vi "Measure Waveform.vi"(6 "Target Data":T1, 8 "error in (no error)":errorcluster, 9 "Measurement":T3, 10 "Channel":T2, 11 "MSOX6004 in":refnum<class "MSOX6004.lvclass">) -> (0 "error out":errorcluster, 2 "Measurement":dbl, 3 "MSOX6004 out":refnum<class "MSOX6004.lvclass">)   [LabVIEW 2018, in "MSOX6004.lvlib" / "MSOX6004.lvclass"]
uses:
  MSOX6004.lvclass
  PPLs/Oscilloscope/Parent/Oscilloscope.lvlibp/Custom Controls/Measurement.ctl
  PPLs/Oscilloscope/Parent/Oscilloscope.lvlibp/Custom Controls/Analog Channels.ctl
  PPLs/Oscilloscope/Parent/Oscilloscope.lvlibp/Custom Controls/Target Data.ctl
  MSOX6004.lvclass/MSOX6004.ctl
  <instrlib>/Keysight InfiniiVision/Keysight InfiniiVision.lvlib
  PPLs/Oscilloscope/Parent/Oscilloscope.lvlibp
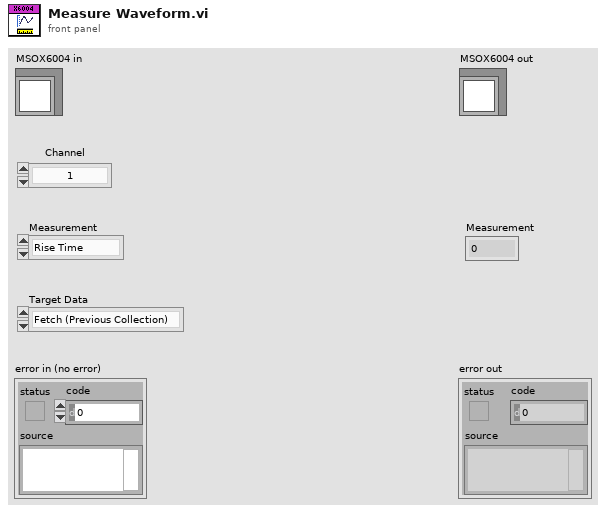
[diagram p1: front panel]
types:
  T1 = typedef "Oscilloscope.lvlibp/Target Data.ctl" = enum16{"Fetch (Previous Collection)", "Measure (New Collection)"}
  T2 = typedef "Oscilloscope.lvlibp/Analog Channels.ctl" = enum16{"1", "2", "3", "4", "5", "6", "7", "8", "9", "10", "11", "12", "13", "14", "15", "16"}
  T3 = typedef "Oscilloscope.lvlibp/Measurement.ctl" = enum16{"Rise Time", "Fall Time", "Frequency", "Period", "RMS (V)", "Peak-Peak (V)", "Max (V)", "Min (V)", "High State (V)", "Low State (V)", "Average (V)", "Width (Negative)", "Width (Positive)", "Duty Cycle (Negative)", "Duty Cycle (Positive)", "Amplitude", "Cycle RMS (V)", "Cycle Avg (V)", "Overshoot", "Preshoot", "Time at Max", "Frequency Counter", "Time at Min", "Delay", "Value at Time", "Phase", "Time at Value", "Time of Edge", "Area", "Burst Width", "Falling Edge Count", "Rising Edge Count", "Falling Pulse Count", "Rising Pulse Count", "Std Dev", "Pulse Width"}
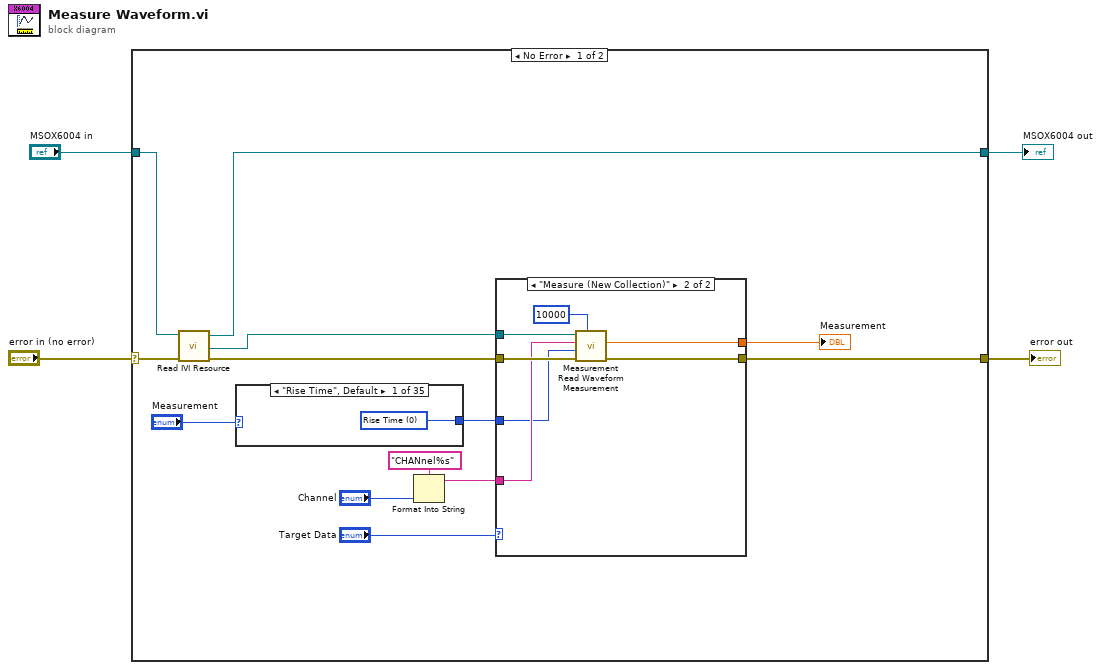
[diagram p0: block diagram]
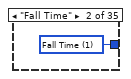
[diagram p2: hidden frame]
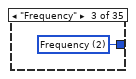
[diagram p3: hidden frame]
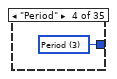
[diagram p4: hidden frame]
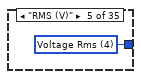
[diagram p5: hidden frame]
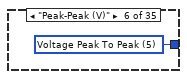
[diagram p6: hidden frame]
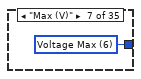
[diagram p7: hidden frame]
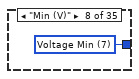
[diagram p8: hidden frame]
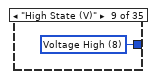
[diagram p9: hidden frame]
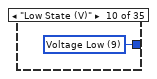
[diagram p10: hidden frame]
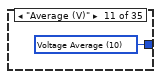
[diagram p11: hidden frame]
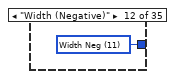
[diagram p12: hidden frame]
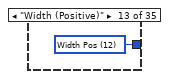
[diagram p13: hidden frame]
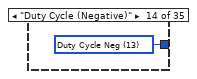
[diagram p14: hidden frame]
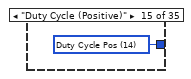
[diagram p15: hidden frame]
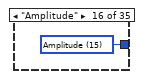
[diagram p16: hidden frame]
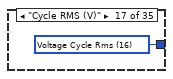
[diagram p17: hidden frame]
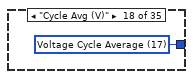
[diagram p18: hidden frame]
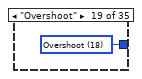
[diagram p19: hidden frame]
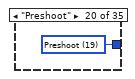
[diagram p20: hidden frame]
diagram:
  n1 = case shown="No Error" "error in (no error)" {
    selector: "error in (no error)" -> [w17 w67]
    tunnel: [w12 w67] -> w3
    tunnel: [w15 w66] -> w2
    tunnel: "MSOX6004 in" -> [w16 w66]
    frame No Error {
      n2 = call "Read IVI Resource.vi"("error in (no error)"=w17, "MSOX6004 in"=w16) -> ("error out"=w13:errorcluster, "IVI Resource"=w10:refnum<k15>, "MSOX6004 out"=w15:refnum<class "MSOX6004.lvclass">)  [unwired: 7 in]
      n3 = case shown="\"Rise Time\", Default" "Measurement" {
        tunnel: [w18 w19 w20 w21 w22 w23 w24 w25 w26 w27 w28 w29 w30 w31 w32 w33 w34 w35 w36 w37 w38 w39 w40 w41 w42 w43 w44 w45 w46 w47 w48 w49 w50 w51 w52] -> w5
        frame "Rise Time", Default {
          w18 = 0 items=["Rise Time"=0, "Fall Time"=1, "Frequency"=2, "Period"=3, "Voltage Rms"=4, "Voltage Peak To Peak"=5, "Voltage Max"=6, "Voltage Min"=7, "Voltage High"=8, "Voltage Low"=9, "Voltage Average"=10, "Width Neg"=11, "Width Pos"=12, "Duty Cycle Neg"=13, "Duty Cycle Pos"=14, "Amplitude"=15, "Voltage Cycle Rms"=16, "Voltage Cycle Average"=17, "Overshoot"=18, "Preshoot"=19, "Measurement Time At Max"=21, "Measurement Frequency Counter"=20, "Measurement Time At Min"=22, "Measurement Delay"=23, "Measurement Value At Time"=25, "Measurement Phase"=24, "Measurement Time At Value"=26, "Measurement Time Of Edge"=27, "Measurement Area"=28, "Measurement Burst Width"=29, "Measurement Falling Edge Count"=30, "Measurement Rising Edge Count"=32, "Measurement Falling Pulse Count"=31, "Measurement Rising Pulse Count"=33, "Measurement Standard Deviation"=34] ("MeasFunction (Rise Time)")
        }
        frame "Fall Time" {
          w19 = 1 items=["Rise Time"=0, "Fall Time"=1, "Frequency"=2, "Period"=3, "Voltage Rms"=4, "Voltage Peak To Peak"=5, "Voltage Max"=6, "Voltage Min"=7, "Voltage High"=8, "Voltage Low"=9, "Voltage Average"=10, "Width Neg"=11, "Width Pos"=12, "Duty Cycle Neg"=13, "Duty Cycle Pos"=14, "Amplitude"=15, "Voltage Cycle Rms"=16, "Voltage Cycle Average"=17, "Overshoot"=18, "Preshoot"=19, "Measurement Time At Max"=21, "Measurement Frequency Counter"=20, "Measurement Time At Min"=22, "Measurement Delay"=23, "Measurement Value At Time"=25, "Measurement Phase"=24, "Measurement Time At Value"=26, "Measurement Time Of Edge"=27, "Measurement Area"=28, "Measurement Burst Width"=29, "Measurement Falling Edge Count"=30, "Measurement Rising Edge Count"=32, "Measurement Falling Pulse Count"=31, "Measurement Rising Pulse Count"=33, "Measurement Standard Deviation"=34] ("MeasFunction (Rise Time)")
        }
        frame "Frequency" {
          w20 = 2 items=["Rise Time"=0, "Fall Time"=1, "Frequency"=2, "Period"=3, "Voltage Rms"=4, "Voltage Peak To Peak"=5, "Voltage Max"=6, "Voltage Min"=7, "Voltage High"=8, "Voltage Low"=9, "Voltage Average"=10, "Width Neg"=11, "Width Pos"=12, "Duty Cycle Neg"=13, "Duty Cycle Pos"=14, "Amplitude"=15, "Voltage Cycle Rms"=16, "Voltage Cycle Average"=17, "Overshoot"=18, "Preshoot"=19, "Measurement Time At Max"=21, "Measurement Frequency Counter"=20, "Measurement Time At Min"=22, "Measurement Delay"=23, "Measurement Value At Time"=25, "Measurement Phase"=24, "Measurement Time At Value"=26, "Measurement Time Of Edge"=27, "Measurement Area"=28, "Measurement Burst Width"=29, "Measurement Falling Edge Count"=30, "Measurement Rising Edge Count"=32, "Measurement Falling Pulse Count"=31, "Measurement Rising Pulse Count"=33, "Measurement Standard Deviation"=34] ("MeasFunction (Rise Time)")
        }
        frame "Period" {
          w21 = 3 items=["Rise Time"=0, "Fall Time"=1, "Frequency"=2, "Period"=3, "Voltage Rms"=4, "Voltage Peak To Peak"=5, "Voltage Max"=6, "Voltage Min"=7, "Voltage High"=8, "Voltage Low"=9, "Voltage Average"=10, "Width Neg"=11, "Width Pos"=12, "Duty Cycle Neg"=13, "Duty Cycle Pos"=14, "Amplitude"=15, "Voltage Cycle Rms"=16, "Voltage Cycle Average"=17, "Overshoot"=18, "Preshoot"=19, "Measurement Time At Max"=21, "Measurement Frequency Counter"=20, "Measurement Time At Min"=22, "Measurement Delay"=23, "Measurement Value At Time"=25, "Measurement Phase"=24, "Measurement Time At Value"=26, "Measurement Time Of Edge"=27, "Measurement Area"=28, "Measurement Burst Width"=29, "Measurement Falling Edge Count"=30, "Measurement Rising Edge Count"=32, "Measurement Falling Pulse Count"=31, "Measurement Rising Pulse Count"=33, "Measurement Standard Deviation"=34] ("MeasFunction (Rise Time)")
        }
        frame "RMS (V)" {
          w22 = 4 items=["Rise Time"=0, "Fall Time"=1, "Frequency"=2, "Period"=3, "Voltage Rms"=4, "Voltage Peak To Peak"=5, "Voltage Max"=6, "Voltage Min"=7, "Voltage High"=8, "Voltage Low"=9, "Voltage Average"=10, "Width Neg"=11, "Width Pos"=12, "Duty Cycle Neg"=13, "Duty Cycle Pos"=14, "Amplitude"=15, "Voltage Cycle Rms"=16, "Voltage Cycle Average"=17, "Overshoot"=18, "Preshoot"=19, "Measurement Time At Max"=21, "Measurement Frequency Counter"=20, "Measurement Time At Min"=22, "Measurement Delay"=23, "Measurement Value At Time"=25, "Measurement Phase"=24, "Measurement Time At Value"=26, "Measurement Time Of Edge"=27, "Measurement Area"=28, "Measurement Burst Width"=29, "Measurement Falling Edge Count"=30, "Measurement Rising Edge Count"=32, "Measurement Falling Pulse Count"=31, "Measurement Rising Pulse Count"=33, "Measurement Standard Deviation"=34] ("MeasFunction (Rise Time)")
        }
        frame "Peak-Peak (V)" {
          w23 = 5 items=["Rise Time"=0, "Fall Time"=1, "Frequency"=2, "Period"=3, "Voltage Rms"=4, "Voltage Peak To Peak"=5, "Voltage Max"=6, "Voltage Min"=7, "Voltage High"=8, "Voltage Low"=9, "Voltage Average"=10, "Width Neg"=11, "Width Pos"=12, "Duty Cycle Neg"=13, "Duty Cycle Pos"=14, "Amplitude"=15, "Voltage Cycle Rms"=16, "Voltage Cycle Average"=17, "Overshoot"=18, "Preshoot"=19, "Measurement Time At Max"=21, "Measurement Frequency Counter"=20, "Measurement Time At Min"=22, "Measurement Delay"=23, "Measurement Value At Time"=25, "Measurement Phase"=24, "Measurement Time At Value"=26, "Measurement Time Of Edge"=27, "Measurement Area"=28, "Measurement Burst Width"=29, "Measurement Falling Edge Count"=30, "Measurement Rising Edge Count"=32, "Measurement Falling Pulse Count"=31, "Measurement Rising Pulse Count"=33, "Measurement Standard Deviation"=34] ("MeasFunction (Rise Time)")
        }
        frame "Max (V)" {
          w24 = 6 items=["Rise Time"=0, "Fall Time"=1, "Frequency"=2, "Period"=3, "Voltage Rms"=4, "Voltage Peak To Peak"=5, "Voltage Max"=6, "Voltage Min"=7, "Voltage High"=8, "Voltage Low"=9, "Voltage Average"=10, "Width Neg"=11, "Width Pos"=12, "Duty Cycle Neg"=13, "Duty Cycle Pos"=14, "Amplitude"=15, "Voltage Cycle Rms"=16, "Voltage Cycle Average"=17, "Overshoot"=18, "Preshoot"=19, "Measurement Time At Max"=21, "Measurement Frequency Counter"=20, "Measurement Time At Min"=22, "Measurement Delay"=23, "Measurement Value At Time"=25, "Measurement Phase"=24, "Measurement Time At Value"=26, "Measurement Time Of Edge"=27, "Measurement Area"=28, "Measurement Burst Width"=29, "Measurement Falling Edge Count"=30, "Measurement Rising Edge Count"=32, "Measurement Falling Pulse Count"=31, "Measurement Rising Pulse Count"=33, "Measurement Standard Deviation"=34] ("MeasFunction (Rise Time)")
        }
        frame "Min (V)" {
          w25 = 7 items=["Rise Time"=0, "Fall Time"=1, "Frequency"=2, "Period"=3, "Voltage Rms"=4, "Voltage Peak To Peak"=5, "Voltage Max"=6, "Voltage Min"=7, "Voltage High"=8, "Voltage Low"=9, "Voltage Average"=10, "Width Neg"=11, "Width Pos"=12, "Duty Cycle Neg"=13, "Duty Cycle Pos"=14, "Amplitude"=15, "Voltage Cycle Rms"=16, "Voltage Cycle Average"=17, "Overshoot"=18, "Preshoot"=19, "Measurement Time At Max"=21, "Measurement Frequency Counter"=20, "Measurement Time At Min"=22, "Measurement Delay"=23, "Measurement Value At Time"=25, "Measurement Phase"=24, "Measurement Time At Value"=26, "Measurement Time Of Edge"=27, "Measurement Area"=28, "Measurement Burst Width"=29, "Measurement Falling Edge Count"=30, "Measurement Rising Edge Count"=32, "Measurement Falling Pulse Count"=31, "Measurement Rising Pulse Count"=33, "Measurement Standard Deviation"=34] ("MeasFunction (Rise Time)")
        }
        frame "High State (V)" {
          w26 = 8 items=["Rise Time"=0, "Fall Time"=1, "Frequency"=2, "Period"=3, "Voltage Rms"=4, "Voltage Peak To Peak"=5, "Voltage Max"=6, "Voltage Min"=7, "Voltage High"=8, "Voltage Low"=9, "Voltage Average"=10, "Width Neg"=11, "Width Pos"=12, "Duty Cycle Neg"=13, "Duty Cycle Pos"=14, "Amplitude"=15, "Voltage Cycle Rms"=16, "Voltage Cycle Average"=17, "Overshoot"=18, "Preshoot"=19, "Measurement Time At Max"=21, "Measurement Frequency Counter"=20, "Measurement Time At Min"=22, "Measurement Delay"=23, "Measurement Value At Time"=25, "Measurement Phase"=24, "Measurement Time At Value"=26, "Measurement Time Of Edge"=27, "Measurement Area"=28, "Measurement Burst Width"=29, "Measurement Falling Edge Count"=30, "Measurement Rising Edge Count"=32, "Measurement Falling Pulse Count"=31, "Measurement Rising Pulse Count"=33, "Measurement Standard Deviation"=34] ("MeasFunction (Rise Time)")
        }
        frame "Low State (V)" {
          w27 = 9 items=["Rise Time"=0, "Fall Time"=1, "Frequency"=2, "Period"=3, "Voltage Rms"=4, "Voltage Peak To Peak"=5, "Voltage Max"=6, "Voltage Min"=7, "Voltage High"=8, "Voltage Low"=9, "Voltage Average"=10, "Width Neg"=11, "Width Pos"=12, "Duty Cycle Neg"=13, "Duty Cycle Pos"=14, "Amplitude"=15, "Voltage Cycle Rms"=16, "Voltage Cycle Average"=17, "Overshoot"=18, "Preshoot"=19, "Measurement Time At Max"=21, "Measurement Frequency Counter"=20, "Measurement Time At Min"=22, "Measurement Delay"=23, "Measurement Value At Time"=25, "Measurement Phase"=24, "Measurement Time At Value"=26, "Measurement Time Of Edge"=27, "Measurement Area"=28, "Measurement Burst Width"=29, "Measurement Falling Edge Count"=30, "Measurement Rising Edge Count"=32, "Measurement Falling Pulse Count"=31, "Measurement Rising Pulse Count"=33, "Measurement Standard Deviation"=34] ("MeasFunction (Rise Time)")
        }
        frame "Average (V)" {
          w28 = 10 items=["Rise Time"=0, "Fall Time"=1, "Frequency"=2, "Period"=3, "Voltage Rms"=4, "Voltage Peak To Peak"=5, "Voltage Max"=6, "Voltage Min"=7, "Voltage High"=8, "Voltage Low"=9, "Voltage Average"=10, "Width Neg"=11, "Width Pos"=12, "Duty Cycle Neg"=13, "Duty Cycle Pos"=14, "Amplitude"=15, "Voltage Cycle Rms"=16, "Voltage Cycle Average"=17, "Overshoot"=18, "Preshoot"=19, "Measurement Time At Max"=21, "Measurement Frequency Counter"=20, "Measurement Time At Min"=22, "Measurement Delay"=23, "Measurement Value At Time"=25, "Measurement Phase"=24, "Measurement Time At Value"=26, "Measurement Time Of Edge"=27, "Measurement Area"=28, "Measurement Burst Width"=29, "Measurement Falling Edge Count"=30, "Measurement Rising Edge Count"=32, "Measurement Falling Pulse Count"=31, "Measurement Rising Pulse Count"=33, "Measurement Standard Deviation"=34] ("MeasFunction (Rise Time)")
        }
        frame "Width (Negative)" {
          w29 = 11 items=["Rise Time"=0, "Fall Time"=1, "Frequency"=2, "Period"=3, "Voltage Rms"=4, "Voltage Peak To Peak"=5, "Voltage Max"=6, "Voltage Min"=7, "Voltage High"=8, "Voltage Low"=9, "Voltage Average"=10, "Width Neg"=11, "Width Pos"=12, "Duty Cycle Neg"=13, "Duty Cycle Pos"=14, "Amplitude"=15, "Voltage Cycle Rms"=16, "Voltage Cycle Average"=17, "Overshoot"=18, "Preshoot"=19, "Measurement Time At Max"=21, "Measurement Frequency Counter"=20, "Measurement Time At Min"=22, "Measurement Delay"=23, "Measurement Value At Time"=25, "Measurement Phase"=24, "Measurement Time At Value"=26, "Measurement Time Of Edge"=27, "Measurement Area"=28, "Measurement Burst Width"=29, "Measurement Falling Edge Count"=30, "Measurement Rising Edge Count"=32, "Measurement Falling Pulse Count"=31, "Measurement Rising Pulse Count"=33, "Measurement Standard Deviation"=34] ("MeasFunction (Rise Time)")
        }
        frame "Width (Positive)" {
          w30 = 12 items=["Rise Time"=0, "Fall Time"=1, "Frequency"=2, "Period"=3, "Voltage Rms"=4, "Voltage Peak To Peak"=5, "Voltage Max"=6, "Voltage Min"=7, "Voltage High"=8, "Voltage Low"=9, "Voltage Average"=10, "Width Neg"=11, "Width Pos"=12, "Duty Cycle Neg"=13, "Duty Cycle Pos"=14, "Amplitude"=15, "Voltage Cycle Rms"=16, "Voltage Cycle Average"=17, "Overshoot"=18, "Preshoot"=19, "Measurement Time At Max"=21, "Measurement Frequency Counter"=20, "Measurement Time At Min"=22, "Measurement Delay"=23, "Measurement Value At Time"=25, "Measurement Phase"=24, "Measurement Time At Value"=26, "Measurement Time Of Edge"=27, "Measurement Area"=28, "Measurement Burst Width"=29, "Measurement Falling Edge Count"=30, "Measurement Rising Edge Count"=32, "Measurement Falling Pulse Count"=31, "Measurement Rising Pulse Count"=33, "Measurement Standard Deviation"=34] ("MeasFunction (Rise Time)")
        }
        frame "Duty Cycle (Negative)" {
          w31 = 13 items=["Rise Time"=0, "Fall Time"=1, "Frequency"=2, "Period"=3, "Voltage Rms"=4, "Voltage Peak To Peak"=5, "Voltage Max"=6, "Voltage Min"=7, "Voltage High"=8, "Voltage Low"=9, "Voltage Average"=10, "Width Neg"=11, "Width Pos"=12, "Duty Cycle Neg"=13, "Duty Cycle Pos"=14, "Amplitude"=15, "Voltage Cycle Rms"=16, "Voltage Cycle Average"=17, "Overshoot"=18, "Preshoot"=19, "Measurement Time At Max"=21, "Measurement Frequency Counter"=20, "Measurement Time At Min"=22, "Measurement Delay"=23, "Measurement Value At Time"=25, "Measurement Phase"=24, "Measurement Time At Value"=26, "Measurement Time Of Edge"=27, "Measurement Area"=28, "Measurement Burst Width"=29, "Measurement Falling Edge Count"=30, "Measurement Rising Edge Count"=32, "Measurement Falling Pulse Count"=31, "Measurement Rising Pulse Count"=33, "Measurement Standard Deviation"=34] ("MeasFunction (Rise Time)")
        }
        frame "Duty Cycle (Positive)" {
          w32 = 14 items=["Rise Time"=0, "Fall Time"=1, "Frequency"=2, "Period"=3, "Voltage Rms"=4, "Voltage Peak To Peak"=5, "Voltage Max"=6, "Voltage Min"=7, "Voltage High"=8, "Voltage Low"=9, "Voltage Average"=10, "Width Neg"=11, "Width Pos"=12, "Duty Cycle Neg"=13, "Duty Cycle Pos"=14, "Amplitude"=15, "Voltage Cycle Rms"=16, "Voltage Cycle Average"=17, "Overshoot"=18, "Preshoot"=19, "Measurement Time At Max"=21, "Measurement Frequency Counter"=20, "Measurement Time At Min"=22, "Measurement Delay"=23, "Measurement Value At Time"=25, "Measurement Phase"=24, "Measurement Time At Value"=26, "Measurement Time Of Edge"=27, "Measurement Area"=28, "Measurement Burst Width"=29, "Measurement Falling Edge Count"=30, "Measurement Rising Edge Count"=32, "Measurement Falling Pulse Count"=31, "Measurement Rising Pulse Count"=33, "Measurement Standard Deviation"=34] ("MeasFunction (Rise Time)")
        }
        frame "Amplitude" {
          w33 = 15 items=["Rise Time"=0, "Fall Time"=1, "Frequency"=2, "Period"=3, "Voltage Rms"=4, "Voltage Peak To Peak"=5, "Voltage Max"=6, "Voltage Min"=7, "Voltage High"=8, "Voltage Low"=9, "Voltage Average"=10, "Width Neg"=11, "Width Pos"=12, "Duty Cycle Neg"=13, "Duty Cycle Pos"=14, "Amplitude"=15, "Voltage Cycle Rms"=16, "Voltage Cycle Average"=17, "Overshoot"=18, "Preshoot"=19, "Measurement Time At Max"=21, "Measurement Frequency Counter"=20, "Measurement Time At Min"=22, "Measurement Delay"=23, "Measurement Value At Time"=25, "Measurement Phase"=24, "Measurement Time At Value"=26, "Measurement Time Of Edge"=27, "Measurement Area"=28, "Measurement Burst Width"=29, "Measurement Falling Edge Count"=30, "Measurement Rising Edge Count"=32, "Measurement Falling Pulse Count"=31, "Measurement Rising Pulse Count"=33, "Measurement Standard Deviation"=34] ("MeasFunction (Rise Time)")
        }
        frame "Cycle RMS (V)" {
          w34 = 16 items=["Rise Time"=0, "Fall Time"=1, "Frequency"=2, "Period"=3, "Voltage Rms"=4, "Voltage Peak To Peak"=5, "Voltage Max"=6, "Voltage Min"=7, "Voltage High"=8, "Voltage Low"=9, "Voltage Average"=10, "Width Neg"=11, "Width Pos"=12, "Duty Cycle Neg"=13, "Duty Cycle Pos"=14, "Amplitude"=15, "Voltage Cycle Rms"=16, "Voltage Cycle Average"=17, "Overshoot"=18, "Preshoot"=19, "Measurement Time At Max"=21, "Measurement Frequency Counter"=20, "Measurement Time At Min"=22, "Measurement Delay"=23, "Measurement Value At Time"=25, "Measurement Phase"=24, "Measurement Time At Value"=26, "Measurement Time Of Edge"=27, "Measurement Area"=28, "Measurement Burst Width"=29, "Measurement Falling Edge Count"=30, "Measurement Rising Edge Count"=32, "Measurement Falling Pulse Count"=31, "Measurement Rising Pulse Count"=33, "Measurement Standard Deviation"=34] ("MeasFunction (Rise Time)")
        }
        frame "Cycle Avg (V)" {
          w35 = 17 items=["Rise Time"=0, "Fall Time"=1, "Frequency"=2, "Period"=3, "Voltage Rms"=4, "Voltage Peak To Peak"=5, "Voltage Max"=6, "Voltage Min"=7, "Voltage High"=8, "Voltage Low"=9, "Voltage Average"=10, "Width Neg"=11, "Width Pos"=12, "Duty Cycle Neg"=13, "Duty Cycle Pos"=14, "Amplitude"=15, "Voltage Cycle Rms"=16, "Voltage Cycle Average"=17, "Overshoot"=18, "Preshoot"=19, "Measurement Time At Max"=21, "Measurement Frequency Counter"=20, "Measurement Time At Min"=22, "Measurement Delay"=23, "Measurement Value At Time"=25, "Measurement Phase"=24, "Measurement Time At Value"=26, "Measurement Time Of Edge"=27, "Measurement Area"=28, "Measurement Burst Width"=29, "Measurement Falling Edge Count"=30, "Measurement Rising Edge Count"=32, "Measurement Falling Pulse Count"=31, "Measurement Rising Pulse Count"=33, "Measurement Standard Deviation"=34] ("MeasFunction (Rise Time)")
        }
        frame "Overshoot" {
          w36 = 18 items=["Rise Time"=0, "Fall Time"=1, "Frequency"=2, "Period"=3, "Voltage Rms"=4, "Voltage Peak To Peak"=5, "Voltage Max"=6, "Voltage Min"=7, "Voltage High"=8, "Voltage Low"=9, "Voltage Average"=10, "Width Neg"=11, "Width Pos"=12, "Duty Cycle Neg"=13, "Duty Cycle Pos"=14, "Amplitude"=15, "Voltage Cycle Rms"=16, "Voltage Cycle Average"=17, "Overshoot"=18, "Preshoot"=19, "Measurement Time At Max"=21, "Measurement Frequency Counter"=20, "Measurement Time At Min"=22, "Measurement Delay"=23, "Measurement Value At Time"=25, "Measurement Phase"=24, "Measurement Time At Value"=26, "Measurement Time Of Edge"=27, "Measurement Area"=28, "Measurement Burst Width"=29, "Measurement Falling Edge Count"=30, "Measurement Rising Edge Count"=32, "Measurement Falling Pulse Count"=31, "Measurement Rising Pulse Count"=33, "Measurement Standard Deviation"=34] ("MeasFunction (Rise Time)")
        }
        frame "Preshoot" {
          w37 = 19 items=["Rise Time"=0, "Fall Time"=1, "Frequency"=2, "Period"=3, "Voltage Rms"=4, "Voltage Peak To Peak"=5, "Voltage Max"=6, "Voltage Min"=7, "Voltage High"=8, "Voltage Low"=9, "Voltage Average"=10, "Width Neg"=11, "Width Pos"=12, "Duty Cycle Neg"=13, "Duty Cycle Pos"=14, "Amplitude"=15, "Voltage Cycle Rms"=16, "Voltage Cycle Average"=17, "Overshoot"=18, "Preshoot"=19, "Measurement Time At Max"=21, "Measurement Frequency Counter"=20, "Measurement Time At Min"=22, "Measurement Delay"=23, "Measurement Value At Time"=25, "Measurement Phase"=24, "Measurement Time At Value"=26, "Measurement Time Of Edge"=27, "Measurement Area"=28, "Measurement Burst Width"=29, "Measurement Falling Edge Count"=30, "Measurement Rising Edge Count"=32, "Measurement Falling Pulse Count"=31, "Measurement Rising Pulse Count"=33, "Measurement Standard Deviation"=34] ("MeasFunction (Rise Time)")
        }
        frame "Time at Max" {
          w38 = 21 items=["Rise Time"=0, "Fall Time"=1, "Frequency"=2, "Period"=3, "Voltage Rms"=4, "Voltage Peak To Peak"=5, "Voltage Max"=6, "Voltage Min"=7, "Voltage High"=8, "Voltage Low"=9, "Voltage Average"=10, "Width Neg"=11, "Width Pos"=12, "Duty Cycle Neg"=13, "Duty Cycle Pos"=14, "Amplitude"=15, "Voltage Cycle Rms"=16, "Voltage Cycle Average"=17, "Overshoot"=18, "Preshoot"=19, "Measurement Time At Max"=21, "Measurement Frequency Counter"=20, "Measurement Time At Min"=22, "Measurement Delay"=23, "Measurement Value At Time"=25, "Measurement Phase"=24, "Measurement Time At Value"=26, "Measurement Time Of Edge"=27, "Measurement Area"=28, "Measurement Burst Width"=29, "Measurement Falling Edge Count"=30, "Measurement Rising Edge Count"=32, "Measurement Falling Pulse Count"=31, "Measurement Rising Pulse Count"=33, "Measurement Standard Deviation"=34] ("MeasFunction (Rise Time)")
        }
        frame "Frequency Counter" {
          w39 = 20 items=["Rise Time"=0, "Fall Time"=1, "Frequency"=2, "Period"=3, "Voltage Rms"=4, "Voltage Peak To Peak"=5, "Voltage Max"=6, "Voltage Min"=7, "Voltage High"=8, "Voltage Low"=9, "Voltage Average"=10, "Width Neg"=11, "Width Pos"=12, "Duty Cycle Neg"=13, "Duty Cycle Pos"=14, "Amplitude"=15, "Voltage Cycle Rms"=16, "Voltage Cycle Average"=17, "Overshoot"=18, "Preshoot"=19, "Measurement Time At Max"=21, "Measurement Frequency Counter"=20, "Measurement Time At Min"=22, "Measurement Delay"=23, "Measurement Value At Time"=25, "Measurement Phase"=24, "Measurement Time At Value"=26, "Measurement Time Of Edge"=27, "Measurement Area"=28, "Measurement Burst Width"=29, "Measurement Falling Edge Count"=30, "Measurement Rising Edge Count"=32, "Measurement Falling Pulse Count"=31, "Measurement Rising Pulse Count"=33, "Measurement Standard Deviation"=34] ("MeasFunction (Rise Time)")
        }
        frame "Time at Min" {
          w40 = 22 items=["Rise Time"=0, "Fall Time"=1, "Frequency"=2, "Period"=3, "Voltage Rms"=4, "Voltage Peak To Peak"=5, "Voltage Max"=6, "Voltage Min"=7, "Voltage High"=8, "Voltage Low"=9, "Voltage Average"=10, "Width Neg"=11, "Width Pos"=12, "Duty Cycle Neg"=13, "Duty Cycle Pos"=14, "Amplitude"=15, "Voltage Cycle Rms"=16, "Voltage Cycle Average"=17, "Overshoot"=18, "Preshoot"=19, "Measurement Time At Max"=21, "Measurement Frequency Counter"=20, "Measurement Time At Min"=22, "Measurement Delay"=23, "Measurement Value At Time"=25, "Measurement Phase"=24, "Measurement Time At Value"=26, "Measurement Time Of Edge"=27, "Measurement Area"=28, "Measurement Burst Width"=29, "Measurement Falling Edge Count"=30, "Measurement Rising Edge Count"=32, "Measurement Falling Pulse Count"=31, "Measurement Rising Pulse Count"=33, "Measurement Standard Deviation"=34] ("MeasFunction (Rise Time)")
        }
        frame "Delay" {
          w41 = 23 items=["Rise Time"=0, "Fall Time"=1, "Frequency"=2, "Period"=3, "Voltage Rms"=4, "Voltage Peak To Peak"=5, "Voltage Max"=6, "Voltage Min"=7, "Voltage High"=8, "Voltage Low"=9, "Voltage Average"=10, "Width Neg"=11, "Width Pos"=12, "Duty Cycle Neg"=13, "Duty Cycle Pos"=14, "Amplitude"=15, "Voltage Cycle Rms"=16, "Voltage Cycle Average"=17, "Overshoot"=18, "Preshoot"=19, "Measurement Time At Max"=21, "Measurement Frequency Counter"=20, "Measurement Time At Min"=22, "Measurement Delay"=23, "Measurement Value At Time"=25, "Measurement Phase"=24, "Measurement Time At Value"=26, "Measurement Time Of Edge"=27, "Measurement Area"=28, "Measurement Burst Width"=29, "Measurement Falling Edge Count"=30, "Measurement Rising Edge Count"=32, "Measurement Falling Pulse Count"=31, "Measurement Rising Pulse Count"=33, "Measurement Standard Deviation"=34] ("MeasFunction (Rise Time)")
        }
        frame "Value at Time" {
          w42 = 25 items=["Rise Time"=0, "Fall Time"=1, "Frequency"=2, "Period"=3, "Voltage Rms"=4, "Voltage Peak To Peak"=5, "Voltage Max"=6, "Voltage Min"=7, "Voltage High"=8, "Voltage Low"=9, "Voltage Average"=10, "Width Neg"=11, "Width Pos"=12, "Duty Cycle Neg"=13, "Duty Cycle Pos"=14, "Amplitude"=15, "Voltage Cycle Rms"=16, "Voltage Cycle Average"=17, "Overshoot"=18, "Preshoot"=19, "Measurement Time At Max"=21, "Measurement Frequency Counter"=20, "Measurement Time At Min"=22, "Measurement Delay"=23, "Measurement Value At Time"=25, "Measurement Phase"=24, "Measurement Time At Value"=26, "Measurement Time Of Edge"=27, "Measurement Area"=28, "Measurement Burst Width"=29, "Measurement Falling Edge Count"=30, "Measurement Rising Edge Count"=32, "Measurement Falling Pulse Count"=31, "Measurement Rising Pulse Count"=33, "Measurement Standard Deviation"=34] ("MeasFunction (Rise Time)")
        }
        frame "Phase" {
          w43 = 24 items=["Rise Time"=0, "Fall Time"=1, "Frequency"=2, "Period"=3, "Voltage Rms"=4, "Voltage Peak To Peak"=5, "Voltage Max"=6, "Voltage Min"=7, "Voltage High"=8, "Voltage Low"=9, "Voltage Average"=10, "Width Neg"=11, "Width Pos"=12, "Duty Cycle Neg"=13, "Duty Cycle Pos"=14, "Amplitude"=15, "Voltage Cycle Rms"=16, "Voltage Cycle Average"=17, "Overshoot"=18, "Preshoot"=19, "Measurement Time At Max"=21, "Measurement Frequency Counter"=20, "Measurement Time At Min"=22, "Measurement Delay"=23, "Measurement Value At Time"=25, "Measurement Phase"=24, "Measurement Time At Value"=26, "Measurement Time Of Edge"=27, "Measurement Area"=28, "Measurement Burst Width"=29, "Measurement Falling Edge Count"=30, "Measurement Rising Edge Count"=32, "Measurement Falling Pulse Count"=31, "Measurement Rising Pulse Count"=33, "Measurement Standard Deviation"=34] ("MeasFunction (Rise Time)")
        }
        frame "Time at Value" {
          w44 = 26 items=["Rise Time"=0, "Fall Time"=1, "Frequency"=2, "Period"=3, "Voltage Rms"=4, "Voltage Peak To Peak"=5, "Voltage Max"=6, "Voltage Min"=7, "Voltage High"=8, "Voltage Low"=9, "Voltage Average"=10, "Width Neg"=11, "Width Pos"=12, "Duty Cycle Neg"=13, "Duty Cycle Pos"=14, "Amplitude"=15, "Voltage Cycle Rms"=16, "Voltage Cycle Average"=17, "Overshoot"=18, "Preshoot"=19, "Measurement Time At Max"=21, "Measurement Frequency Counter"=20, "Measurement Time At Min"=22, "Measurement Delay"=23, "Measurement Value At Time"=25, "Measurement Phase"=24, "Measurement Time At Value"=26, "Measurement Time Of Edge"=27, "Measurement Area"=28, "Measurement Burst Width"=29, "Measurement Falling Edge Count"=30, "Measurement Rising Edge Count"=32, "Measurement Falling Pulse Count"=31, "Measurement Rising Pulse Count"=33, "Measurement Standard Deviation"=34] ("MeasFunction (Rise Time)")
        }
        frame "Time of Edge" {
          w45 = 27 items=["Rise Time"=0, "Fall Time"=1, "Frequency"=2, "Period"=3, "Voltage Rms"=4, "Voltage Peak To Peak"=5, "Voltage Max"=6, "Voltage Min"=7, "Voltage High"=8, "Voltage Low"=9, "Voltage Average"=10, "Width Neg"=11, "Width Pos"=12, "Duty Cycle Neg"=13, "Duty Cycle Pos"=14, "Amplitude"=15, "Voltage Cycle Rms"=16, "Voltage Cycle Average"=17, "Overshoot"=18, "Preshoot"=19, "Measurement Time At Max"=21, "Measurement Frequency Counter"=20, "Measurement Time At Min"=22, "Measurement Delay"=23, "Measurement Value At Time"=25, "Measurement Phase"=24, "Measurement Time At Value"=26, "Measurement Time Of Edge"=27, "Measurement Area"=28, "Measurement Burst Width"=29, "Measurement Falling Edge Count"=30, "Measurement Rising Edge Count"=32, "Measurement Falling Pulse Count"=31, "Measurement Rising Pulse Count"=33, "Measurement Standard Deviation"=34] ("MeasFunction (Rise Time)")
        }
        frame "Area" {
          w46 = 28 items=["Rise Time"=0, "Fall Time"=1, "Frequency"=2, "Period"=3, "Voltage Rms"=4, "Voltage Peak To Peak"=5, "Voltage Max"=6, "Voltage Min"=7, "Voltage High"=8, "Voltage Low"=9, "Voltage Average"=10, "Width Neg"=11, "Width Pos"=12, "Duty Cycle Neg"=13, "Duty Cycle Pos"=14, "Amplitude"=15, "Voltage Cycle Rms"=16, "Voltage Cycle Average"=17, "Overshoot"=18, "Preshoot"=19, "Measurement Time At Max"=21, "Measurement Frequency Counter"=20, "Measurement Time At Min"=22, "Measurement Delay"=23, "Measurement Value At Time"=25, "Measurement Phase"=24, "Measurement Time At Value"=26, "Measurement Time Of Edge"=27, "Measurement Area"=28, "Measurement Burst Width"=29, "Measurement Falling Edge Count"=30, "Measurement Rising Edge Count"=32, "Measurement Falling Pulse Count"=31, "Measurement Rising Pulse Count"=33, "Measurement Standard Deviation"=34] ("MeasFunction (Rise Time)")
        }
        frame "Burst Width" {
          w47 = 29 items=["Rise Time"=0, "Fall Time"=1, "Frequency"=2, "Period"=3, "Voltage Rms"=4, "Voltage Peak To Peak"=5, "Voltage Max"=6, "Voltage Min"=7, "Voltage High"=8, "Voltage Low"=9, "Voltage Average"=10, "Width Neg"=11, "Width Pos"=12, "Duty Cycle Neg"=13, "Duty Cycle Pos"=14, "Amplitude"=15, "Voltage Cycle Rms"=16, "Voltage Cycle Average"=17, "Overshoot"=18, "Preshoot"=19, "Measurement Time At Max"=21, "Measurement Frequency Counter"=20, "Measurement Time At Min"=22, "Measurement Delay"=23, "Measurement Value At Time"=25, "Measurement Phase"=24, "Measurement Time At Value"=26, "Measurement Time Of Edge"=27, "Measurement Area"=28, "Measurement Burst Width"=29, "Measurement Falling Edge Count"=30, "Measurement Rising Edge Count"=32, "Measurement Falling Pulse Count"=31, "Measurement Rising Pulse Count"=33, "Measurement Standard Deviation"=34] ("MeasFunction (Rise Time)")
        }
        frame "Falling Edge Count" {
          w48 = 30 items=["Rise Time"=0, "Fall Time"=1, "Frequency"=2, "Period"=3, "Voltage Rms"=4, "Voltage Peak To Peak"=5, "Voltage Max"=6, "Voltage Min"=7, "Voltage High"=8, "Voltage Low"=9, "Voltage Average"=10, "Width Neg"=11, "Width Pos"=12, "Duty Cycle Neg"=13, "Duty Cycle Pos"=14, "Amplitude"=15, "Voltage Cycle Rms"=16, "Voltage Cycle Average"=17, "Overshoot"=18, "Preshoot"=19, "Measurement Time At Max"=21, "Measurement Frequency Counter"=20, "Measurement Time At Min"=22, "Measurement Delay"=23, "Measurement Value At Time"=25, "Measurement Phase"=24, "Measurement Time At Value"=26, "Measurement Time Of Edge"=27, "Measurement Area"=28, "Measurement Burst Width"=29, "Measurement Falling Edge Count"=30, "Measurement Rising Edge Count"=32, "Measurement Falling Pulse Count"=31, "Measurement Rising Pulse Count"=33, "Measurement Standard Deviation"=34] ("MeasFunction (Rise Time)")
        }
        frame "Rising Edge Count" {
          w49 = 32 items=["Rise Time"=0, "Fall Time"=1, "Frequency"=2, "Period"=3, "Voltage Rms"=4, "Voltage Peak To Peak"=5, "Voltage Max"=6, "Voltage Min"=7, "Voltage High"=8, "Voltage Low"=9, "Voltage Average"=10, "Width Neg"=11, "Width Pos"=12, "Duty Cycle Neg"=13, "Duty Cycle Pos"=14, "Amplitude"=15, "Voltage Cycle Rms"=16, "Voltage Cycle Average"=17, "Overshoot"=18, "Preshoot"=19, "Measurement Time At Max"=21, "Measurement Frequency Counter"=20, "Measurement Time At Min"=22, "Measurement Delay"=23, "Measurement Value At Time"=25, "Measurement Phase"=24, "Measurement Time At Value"=26, "Measurement Time Of Edge"=27, "Measurement Area"=28, "Measurement Burst Width"=29, "Measurement Falling Edge Count"=30, "Measurement Rising Edge Count"=32, "Measurement Falling Pulse Count"=31, "Measurement Rising Pulse Count"=33, "Measurement Standard Deviation"=34] ("MeasFunction (Rise Time)")
        }
        frame "Falling Pulse Count" {
          w50 = 31 items=["Rise Time"=0, "Fall Time"=1, "Frequency"=2, "Period"=3, "Voltage Rms"=4, "Voltage Peak To Peak"=5, "Voltage Max"=6, "Voltage Min"=7, "Voltage High"=8, "Voltage Low"=9, "Voltage Average"=10, "Width Neg"=11, "Width Pos"=12, "Duty Cycle Neg"=13, "Duty Cycle Pos"=14, "Amplitude"=15, "Voltage Cycle Rms"=16, "Voltage Cycle Average"=17, "Overshoot"=18, "Preshoot"=19, "Measurement Time At Max"=21, "Measurement Frequency Counter"=20, "Measurement Time At Min"=22, "Measurement Delay"=23, "Measurement Value At Time"=25, "Measurement Phase"=24, "Measurement Time At Value"=26, "Measurement Time Of Edge"=27, "Measurement Area"=28, "Measurement Burst Width"=29, "Measurement Falling Edge Count"=30, "Measurement Rising Edge Count"=32, "Measurement Falling Pulse Count"=31, "Measurement Rising Pulse Count"=33, "Measurement Standard Deviation"=34] ("MeasFunction (Rise Time)")
        }
        frame "Rising Pulse Count" {
          w51 = 33 items=["Rise Time"=0, "Fall Time"=1, "Frequency"=2, "Period"=3, "Voltage Rms"=4, "Voltage Peak To Peak"=5, "Voltage Max"=6, "Voltage Min"=7, "Voltage High"=8, "Voltage Low"=9, "Voltage Average"=10, "Width Neg"=11, "Width Pos"=12, "Duty Cycle Neg"=13, "Duty Cycle Pos"=14, "Amplitude"=15, "Voltage Cycle Rms"=16, "Voltage Cycle Average"=17, "Overshoot"=18, "Preshoot"=19, "Measurement Time At Max"=21, "Measurement Frequency Counter"=20, "Measurement Time At Min"=22, "Measurement Delay"=23, "Measurement Value At Time"=25, "Measurement Phase"=24, "Measurement Time At Value"=26, "Measurement Time Of Edge"=27, "Measurement Area"=28, "Measurement Burst Width"=29, "Measurement Falling Edge Count"=30, "Measurement Rising Edge Count"=32, "Measurement Falling Pulse Count"=31, "Measurement Rising Pulse Count"=33, "Measurement Standard Deviation"=34] ("MeasFunction (Rise Time)")
        }
        frame "Std Dev" {
          w52 = 34 items=["Rise Time"=0, "Fall Time"=1, "Frequency"=2, "Period"=3, "Voltage Rms"=4, "Voltage Peak To Peak"=5, "Voltage Max"=6, "Voltage Min"=7, "Voltage High"=8, "Voltage Low"=9, "Voltage Average"=10, "Width Neg"=11, "Width Pos"=12, "Duty Cycle Neg"=13, "Duty Cycle Pos"=14, "Amplitude"=15, "Voltage Cycle Rms"=16, "Voltage Cycle Average"=17, "Overshoot"=18, "Preshoot"=19, "Measurement Time At Max"=21, "Measurement Frequency Counter"=20, "Measurement Time At Min"=22, "Measurement Delay"=23, "Measurement Value At Time"=25, "Measurement Phase"=24, "Measurement Time At Value"=26, "Measurement Time Of Edge"=27, "Measurement Area"=28, "Measurement Burst Width"=29, "Measurement Falling Edge Count"=30, "Measurement Rising Edge Count"=32, "Measurement Falling Pulse Count"=31, "Measurement Rising Pulse Count"=33, "Measurement Standard Deviation"=34] ("MeasFunction (Rise Time)")
        }
      }
      n4 = Format Into String(format string="CHANnel%s", "Channel") -> (resulting string=w7:string)  [unwired: 2 in, 1 out]
      n5 = case shown="\"Measure (New Collection)\"" "Target Data" {
        tunnel: w13 -> [w57 w65]
        tunnel: [w55 w64] -> w12
        tunnel: [w56 w63] -> w11
        tunnel: w10 -> [w58 w62]
        tunnel: w7 -> [w53 w61]
        tunnel: w5 -> [w54 w60]
        frame "Fetch (Previous Collection)", Default {
          n6 = call <instrlib>:"Measurement Fetch Waveform Measurement.vi"("error in (no error)"=w57, "MeasFunction (Rise Time)"=w54, "Measurement2"=w53, "instrument handle"=w58) -> ("error out"=w55:errorcluster, "Measurement"=w56:dbl)  [unwired: 5 in, 1 out]
        }
        frame "Measure (New Collection)" {
          n7 = call <instrlib>:"Measurement Read Waveform Measurement.vi"("MaxTimeMilliseconds"=10000, "error in (no error)"=w65, "MeasFunction (Rise Time)"=w60, "Measurement2"=w61, "instrument handle"=w62) -> ("error out"=w64:errorcluster, "Measurement"=w63:dbl)  [unwired: 4 in, 1 out]
        }
      }
      "Measurement" <- w11
    }
    frame Error {
    }
  }
  "error out" <- w3
  "MSOX6004 out" <- w2
